vi "Get Ticks.vi"() -> (0 "Tick Count(Ticks)":u32)   [LabVIEW 2019]
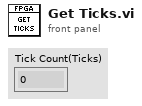
[diagram p1: front panel]
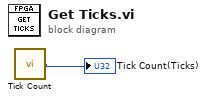
[diagram p0: block diagram]
diagram:
  n1 = call "Tick Count"() -> ("Tick Count(Ticks)"=→"Tick Count(Ticks)":u32)
